vi "ringBuffer.vi"(0 "Utilities in":refnum<class "Utilities.lvclass">, 1 "size":i32=3, 5 "val":dbl=2.0 format="%#_13g", 7 "operation":T1, 11 "error in (no error)":errorcluster) -> (4 "Utilities out":refnum<class "Utilities.lvclass">, 6 "buffer out":dbl[](array[numeric]), 15 "error out":errorcluster)   [LabVIEW 2021, in "Utilities.lvclass"]
uses:
  Utilities.lvclass
  ringBufferCommands.ctl
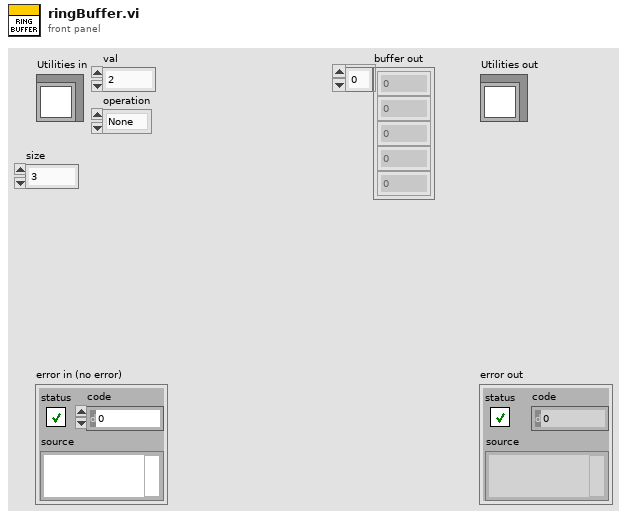
[diagram p1: front panel]
types:
  T1 = typedef "ringBufferCommands.ctl" = enum16{"None", "Push", "Pop"}
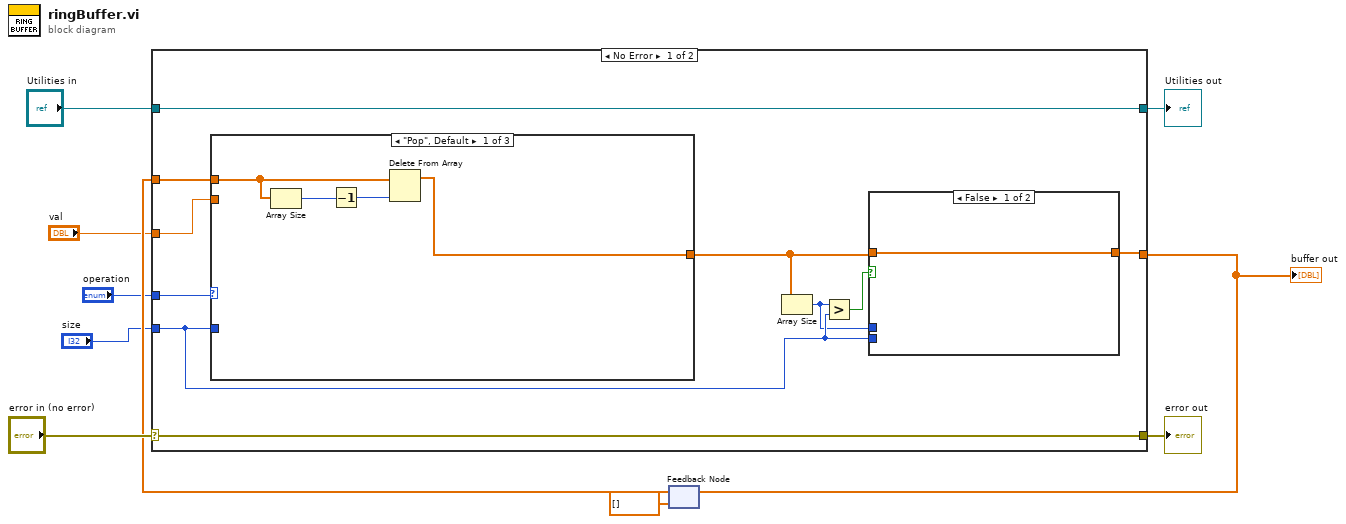
[diagram p0: block diagram]
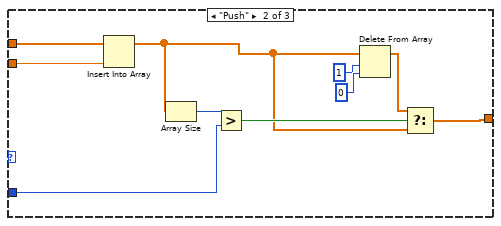
[diagram p2: hidden frame]
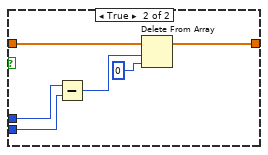
[diagram p4: hidden frame]
diagram:
  n1 = feedback #1(dbl[] []) -> (w6:dbl[])
  n2 = case shown="No Error" "error in (no error)" {
    selector: "error in (no error)" -> [w19 w44]
    tunnel: [w19 w44] -> w9
    tunnel: [w20 w43] -> w7
    tunnel: "Utilities in" -> [w20 w43]
    tunnel: w6 -> [w18 _]
    tunnel: "val" -> [w17 _]
    tunnel: [w14 _] -> w4
    tunnel: "size" -> [w13 _]
    tunnel: "operation" -> [w11 _]
    frame No Error {
      n3 = case shown="\"Pop\", Default" w11 {
        tunnel: w18 -> [w23 w34 w35]
        tunnel: w17 -> [_ w33 _]
        tunnel: [w24 w26 w35] -> w15
        tunnel: w13 -> [_ w31 _]
        frame "Pop", Default {
          n4 = Array Size(array=w23) -> (size(s)=w22:i32)
          n5 = Decrement(x=w22) -> (x-1=w21:i32)
          n6 = Delete From Array(array=w23, index=w21) -> (array with subset deleted=w24:dbl[])  [unwired: 1 in, 1 out]
        }
        frame "Push" {
          n7 = Insert Into Array(array=w34, new element=w33) -> (w27:dbl[])  [unwired: 1 in]
          n8 = Array Size(array=w27) -> (size(s)=w32:i32)
          n9 = Greater?(x=w32, y=w31) -> (0:w30:bool)
          n10 = Delete From Array(array=w27, length=1, index=0) -> (array with subset deleted=w25:dbl[])  [unwired: 1 out]
          n11 = Select(t=w25, s=w30, f=w27) -> (s? t:f=w26:dbl[])
        }
        frame "None" {
        }
      }
      n12 = Array Size(array=w15) -> (size(s)=w12:i32)
      n13 = Greater?(x=w12, y=w13) -> (0:w16:bool)
      n14 = case shown="False" w16 {
        tunnel: w15 -> [w36 w42]
        tunnel: [w36 w37] -> w14
        tunnel: w13 -> [_ w39]
        tunnel: w12 -> [_ w40]
        frame False {
        }
        frame True {
          n15 = Subtract(x=w40, y=w39) -> (x-y=w38:i32)
          n16 = Delete From Array(array=w42, length=w38, index=0) -> (array with subset deleted=w37:dbl[])  [unwired: 1 out]
        }
      }
    }
    frame Error {
    }
  }
  "error out" <- w9
  "Utilities out" <- w7
  "buffer out" <- w4
  n17 = feedback-in #1(w4) -> ()
